vi "IngresoDePoc.vi"() -> ()   [LabVIEW 2012]
uses:
  <vilib>/addons/database/Auxilliary.llb/DB Tools Parameter Info.ctl
  <vilib>/addons/database/Auxilliary.llb/DB Tools DataTypes.ctl
  <vilib>/addons/database/Auxilliary.llb/DB Tools Parameter Dir.ctl
  <vilib>/addons/database/Connection.llb/DB Tools Open Connec (Path).vi
  <vilib>/addons/database/Command.llb/Cmd Set Parameter Value (C).vi
  <vilib>/addons/database/Command.llb/Cmd Execute.vi
  <vilib>/addons/database/Recordset.llb/Rec Destroy - Command.vi
  <vilib>/addons/database/Command.llb/Cmd Delete.vi
  <vilib>/addons/database/NI_Database_API.lvlib
panel:
  in  "Password":string
  in  "Marca":string
  in  "Numero de SIM":string
  in  "Imei":string
  in  "Ciudad":string
  in  "Numero del Propietario":string
  in  "Dirección":string
  in  "Razón Social":string
  in  "Propietario":string
  in  "Icono":string
  in  "Numero de la Ruta":string
  in  "Ruta":string
  out "Auditor Producto":string[](array[string])
  in  "A P":bool
  out "Auditor Servicio Técnico":string[](array[string])
  in  "A ST":bool
  in  "OK":bool
  in  "stop":bool
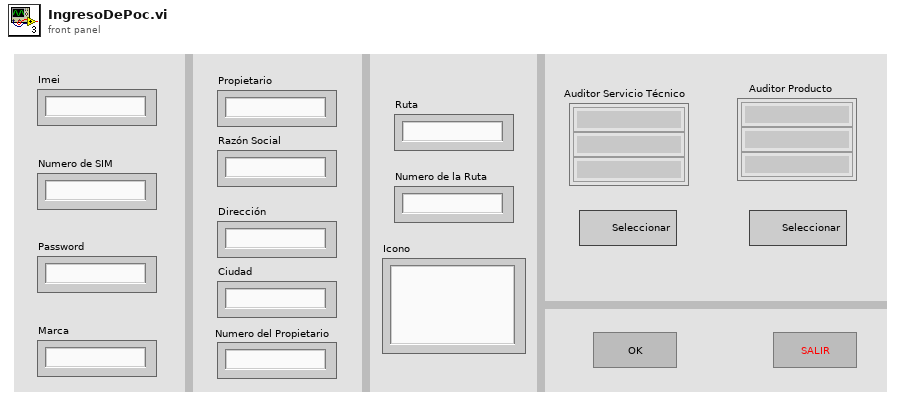
[diagram p1: front panel]
types:
  T1 = typedef "NI_Database_API.lvlib/DB Tools Parameter Info.ctl" = cluster{"parameter name":string, "type":T2, "direction":T3, "value":variant}
  T2 = typedef "NI_Database_API.lvlib/DB Tools DataTypes.ctl" = enum16{"String", "Long (I32)", "Single (SGL)", "Double (DBL)", "Date/Time", "Binary"}
  T3 = typedef "NI_Database_API.lvlib/DB Tools Parameter Dir.ctl" = enum32{"Input", "Output", "Input/Output", "Return Value"}
  T4 = typedef "NI_Database_API.lvlib/Conn ObjectReference.ctl" = refnum<k1>
  T5 = typedef "NI_Database_API.lvlib/Cmd ObjectReference.ctl" = refnum<k1>
  T6 = typedef "NI_Database_API.lvlib/Cmd-Rec Object Reference.ctl" = refnum<k1>
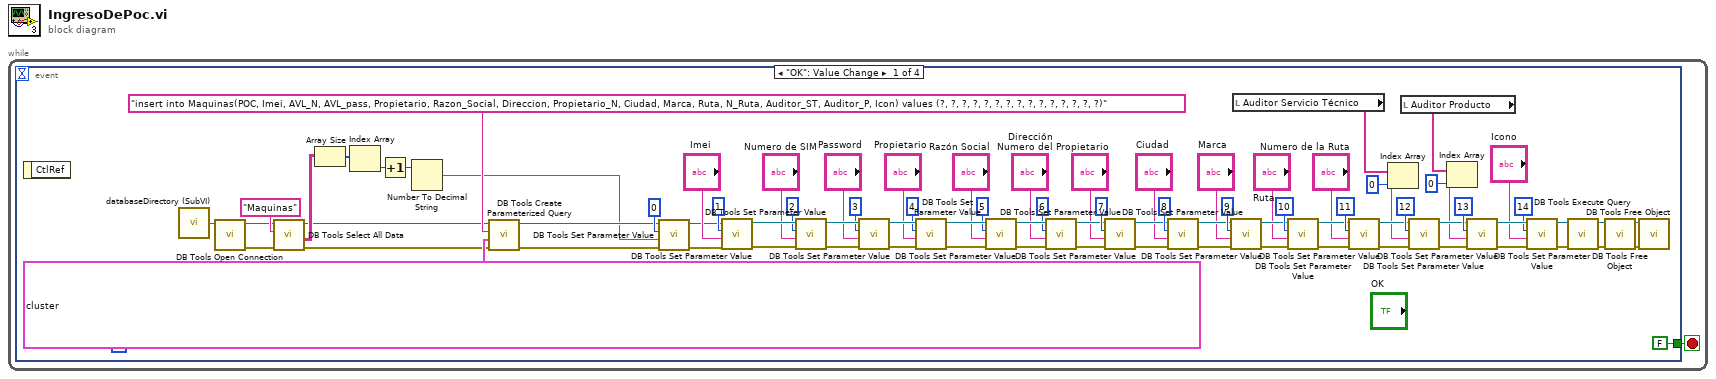
[diagram p0: block diagram]
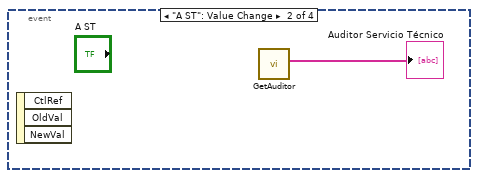
[diagram p2: hidden frame]
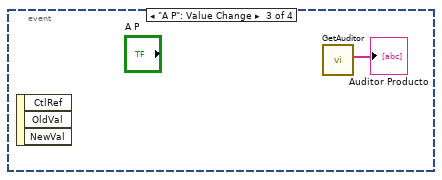
[diagram p3: hidden frame]
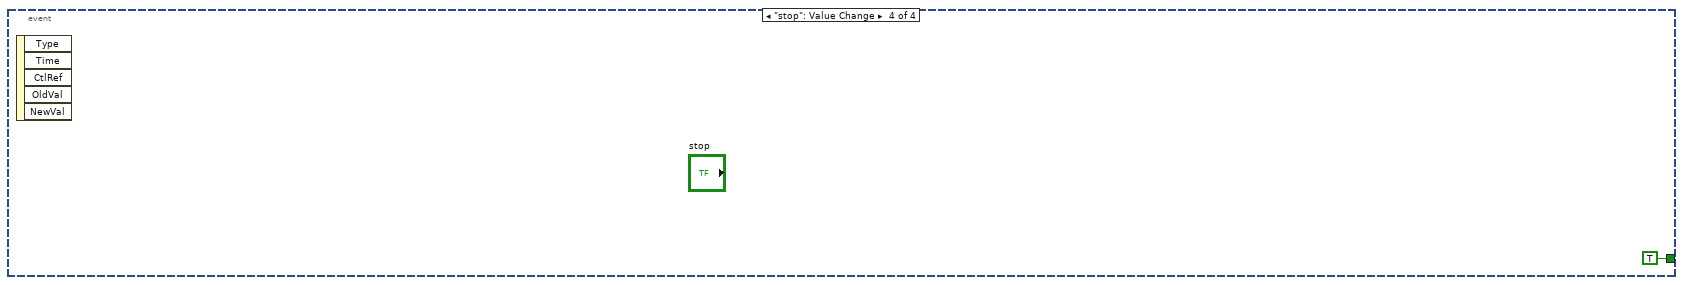
[diagram p4: hidden frame]
diagram:
  n1 = while {
    stop <- w1 stop-if-true
    n2 = event shown="[0] \"OK\": Value Change" {
      selector: _ -> [_ _ _ _]
      dyn-events: _ -> [_ _ _ _]
      timeout: _ -> [_ _ _ _]
      tunnel: [FALSE _ _ TRUE] -> w1
      event "OK": Value Change {
        n3 = event-data() -> ()  [unwired: 1 in, 1 out]
        n4 = call "databaseDirectory (SubVI).vi"() -> ("Application Directory"=w66:path)  [unwired: 1 in]
        n5 = call-poly <vilib>:"DB Tools Open Connection.vi"("connection information"=w66) -> ("error out"=w18:errorcluster, "connection reference"=w17:T4)  [unwired: 7 in]
        n6 = call <vilib>:"DB Tools Select All Data.vi"("error in (no error)"=w18, "table"="Maquinas", "connection reference"=w17) -> ("error out"=w21:errorcluster, "data"=w23:string[][], "connection reference out"=w20:T4)  [unwired: 3 in]
        n7 = Array Size(array=w23) -> (size(s)=w22:i32[])
        n8 = Index Array(array=w22) -> (element=w9:i32)  [unwired: 1 in]
        n9 = Increment(x=w9) -> (x+1=w10:i32)
        n10 = Number To Decimal String(number=w10) -> (decimal integer string=w11:string)  [unwired: 1 in]
        n11 = call <vilib>:"DB Tools Create Parameterized Query.vi"("error in (no error)"=w21, "parameters"=T1[] [{"parameter name"="POC", "type"=enum."String", "direction"=enum."Input", "value"=variant}, {"parameter name"="Imei", "type"=enum."String", "direction"=enum."Input", "value"=variant}, {"parameter name"="AVL_N", "type"=enum."String", "direction"=enum."Input", "value"=variant}, {"parameter name"="AVL_pass", "type"=enum."String", "direction"=enum."Input", "value"=variant}, {"parameter name"="Propietario", "type"=enum."String", "direction"=enum."Input", "value"=variant}, {"parameter name"="Razon_Social", "type"=enum."String", "direction"=enum."Input", "value"=variant}, {"parameter name"="Direccion", "type"=enum."String", "direction"=enum."Input", "value"=variant}, {"parameter name"="Propietario_N", "type"=enum."String", "direction"=enum."Input", "value"=variant}, {"parameter name"="Ciudad", "type"=enum."String", "direction"=enum."Input", "value"=variant}, {"parameter name"="Marca", "type"=enum."String", "direction"=enum."Input", "value"=variant}, {"parameter name"="Ruta", "type"=enum."String", "direction"=enum."Input", "value"=variant}, {"parameter name"="N_Ruta", "type"=enum."String", "direction"=enum."Input", "value"=variant}, {"parameter name"="Auditor_ST", "type"=enum."Single (SGL)", "direction"=enum."Input", "value"=variant}, {"parameter name"="Auditor_P", "type"=enum."Single (SGL)", "direction"=enum."Input", "value"=variant}, {"parameter name"="Icon", "type"=enum."String", "direction"=enum."Input", "value"=variant}], "SQL query"="insert into Maquinas(POC, Imei, AVL_N, AVL_pass, Propietario, Razon_Social, Direccion, Propietario_N, Ciudad, Marca, Ruta, N_Ruta, Auditor_ST, Auditor_P, Icon) values (?, ?, ?, ?, ?, ?, ?, ?, ?, ?, ?, ?, ?, ?, ?)", "connection reference"=w20) -> ("error out"=w14:errorcluster, "command reference"=w15:T5)  [unwired: 3 in, 1 out]
        n12 = call-poly <vilib>:"DB Tools Set Parameter Value.vi"("error in (no error)"=w14, "value"=w11, "parameter index"=0, "command reference"=w15) -> ("error out"=w13:errorcluster, "command reference out"=w12:T5)  [unwired: 4 in]
        n13 = call-poly <vilib>:"DB Tools Set Parameter Value.vi"("error in (no error)"=w13, "value"="Imei", "parameter index"=1, "command reference"=w12) -> ("error out"=w84:errorcluster, "command reference out"=w83:T5)  [unwired: 4 in]
        n14 = call-poly <vilib>:"DB Tools Set Parameter Value.vi"("error in (no error)"=w84, "value"="Numero de SIM", "parameter index"=2, "command reference"=w83) -> ("error out"=w82:errorcluster, "command reference out"=w81:T5)  [unwired: 4 in]
        n15 = call-poly <vilib>:"DB Tools Set Parameter Value.vi"("error in (no error)"=w82, "value"="Password", "parameter index"=3, "command reference"=w81) -> ("error out"=w75:errorcluster, "command reference out"=w74:T5)  [unwired: 4 in]
        n16 = call-poly <vilib>:"DB Tools Set Parameter Value.vi"("error in (no error)"=w75, "value"="Propietario", "parameter index"=4, "command reference"=w74) -> ("error out"=w76:errorcluster, "command reference out"=w77:T5)  [unwired: 4 in]
        n17 = call-poly <vilib>:"DB Tools Set Parameter Value.vi"("error in (no error)"=w76, "value"="Razón Social", "parameter index"=5, "command reference"=w77) -> ("error out"=w72:errorcluster, "command reference out"=w73:T5)  [unwired: 4 in]
        n18 = call-poly <vilib>:"DB Tools Set Parameter Value.vi"("error in (no error)"=w72, "value"="Dirección", "parameter index"=6, "command reference"=w73) -> ("error out"=w45:errorcluster, "command reference out"=w46:T5)  [unwired: 4 in]
        n19 = call-poly <vilib>:"DB Tools Set Parameter Value.vi"("error in (no error)"=w45, "value"="Numero del Propietario", "parameter index"=7, "command reference"=w46) -> ("error out"=w44:errorcluster, "command reference out"=w47:T5)  [unwired: 4 in]
        n20 = call-poly <vilib>:"DB Tools Set Parameter Value.vi"("error in (no error)"=w44, "value"="Ciudad", "parameter index"=8, "command reference"=w47) -> ("error out"=w43:errorcluster, "command reference out"=w48:T5)  [unwired: 4 in]
        n21 = call-poly <vilib>:"DB Tools Set Parameter Value.vi"("error in (no error)"=w43, "value"="Marca", "parameter index"=9, "command reference"=w48) -> ("error out"=w42:errorcluster, "command reference out"=w50:T5)  [unwired: 4 in]
        n22 = local read "Auditor Servicio Técnico"() -> (w7:string[])
        n23 = call-poly <vilib>:"DB Tools Set Parameter Value.vi"("error in (no error)"=w42, "value"="Ruta", "parameter index"=10, "command reference"=w50) -> ("error out"=w41:errorcluster, "command reference out"=w49:T5)  [unwired: 4 in]
        n24 = call-poly <vilib>:"DB Tools Set Parameter Value.vi"("error in (no error)"=w41, "value"="Numero de la Ruta", "parameter index"=11, "command reference"=w49) -> ("error out"=w40:errorcluster, "command reference out"=w51:T5)  [unwired: 4 in]
        n25 = Index Array(array=w7, index=0) -> (element=w6:string)
        n26 = local read "Auditor Producto"() -> (w4:string[])
        n27 = call-poly <vilib>:"DB Tools Set Parameter Value.vi"("error in (no error)"=w40, "value"=w6, "parameter index"=12, "command reference"=w51) -> ("error out"=w29:errorcluster, "command reference out"=w30:T5)  [unwired: 4 in]
        n28 = Index Array(array=w4, index=0) -> (element=w5:string)
        n29 = call-poly <vilib>:"DB Tools Set Parameter Value.vi"("error in (no error)"=w29, "value"=w5, "parameter index"=13, "command reference"=w30) -> ("error out"=w34:errorcluster, "command reference out"=w33:T5)  [unwired: 4 in]
        n30 = call-poly <vilib>:"DB Tools Set Parameter Value.vi"("error in (no error)"=w34, "value"="Icono", "parameter index"=14, "command reference"=w33) -> ("error out"=w28:errorcluster, "command reference out"=w27:T5)  [unwired: 4 in]
        n31 = call-poly <vilib>:"DB Tools Execute Query.vi"("error in (no error)"=w28, "command reference"=w27) -> ("error out"=w80:errorcluster, "command-recordset reference"=w79:T6)  [unwired: 6 in]
        n32 = call-poly <vilib>:"DB Tools Free Object.vi"("error in (no error)"=w80, "command-recordset reference"=w79) -> ("error out"=w78:errorcluster, "command reference"=w26:T5)  [unwired: 8 in]
        n33 = call-poly <vilib>:"DB Tools Free Object.vi"("error in (no error)"=w78, "command reference"=w26) -> ()  [unwired: 8 in, 2 out]
      }
      event "A ST": Value Change {
        n34 = event-data() -> ()  [unwired: 1 in, 3 out]
        n35 = call "GetAuditor.vi"() -> ("Array"=→"Auditor Servicio Técnico":string[])  [unwired: 11 in]
      }
      event "A P": Value Change {
        n36 = event-data() -> ()  [unwired: 1 in, 3 out]
        n37 = call "GetAuditor.vi"() -> ("Array"=→"Auditor Producto":string[])  [unwired: 11 in]
      }
      event "stop": Value Change {
        n38 = event-data() -> ()  [unwired: 1 in, 5 out]
      }
    }
  }
